vi "FTW-CodeGen-Prototype.vi"(0 "REPLACED_Connection":refnum<k24>, 2 "REPLACED_SQL Script":string, 5 "ADAPT_Data to Insert":T1(array[cluster]), 11 "REPLACED_error in":errorcluster) -> (4 "REPLACED_Connection out":refnum<k24>, 8 "REPLACED_Time to Execute":dbl format="%.6fsec", 10 "REPLACED_Number of Rows Inserted":i32, 15 "REPLACED_error out":errorcluster)   [LabVIEW 2015, in "FTW-dotNet-SQL-Insert.xnode"]
uses:
  FTW-dotNet-SQL-Insert.xnode
  System.Data
  src/error/FTW-ERR-ThrowError.vi
  src/error/FTW-ERR-CallChain.vi
  src/string/FTW-STR-ReplaceWhitespace.vi
  src/string/FTW-STR-Array-Delimit.vi
panel:
  # "Inputs"
  # "Outputs"
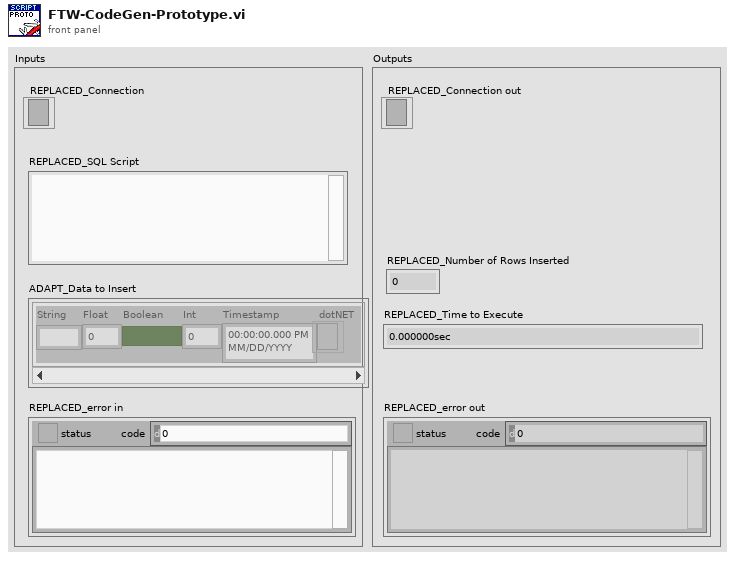
[diagram p1: front panel]
types:
  T1 = cluster{"String":string, "Float":dbl, "Boolean":bool, "Int":i64, "Timestamp":timestamp, "dotNET":refnum<k24>}[]
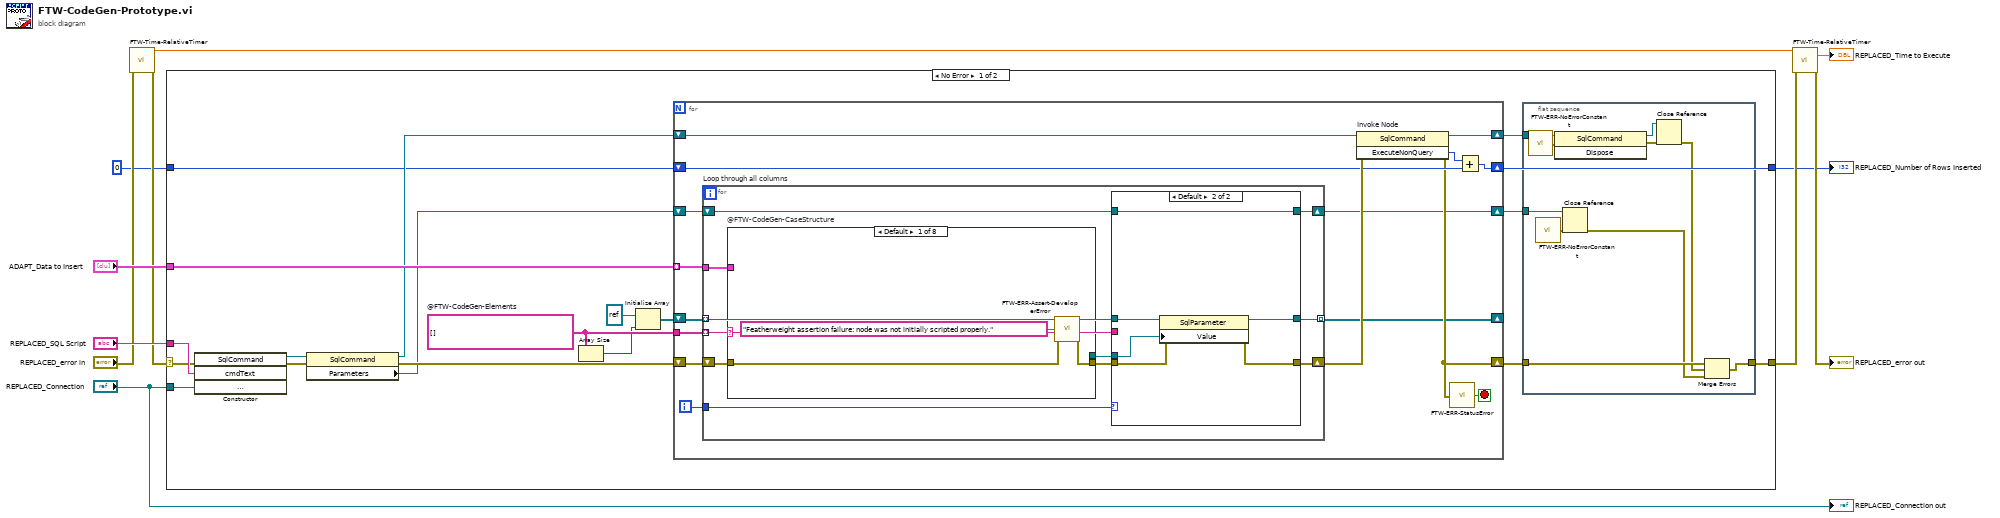
[diagram p0: block diagram]
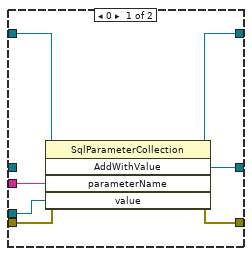
[diagram p2: hidden frame]
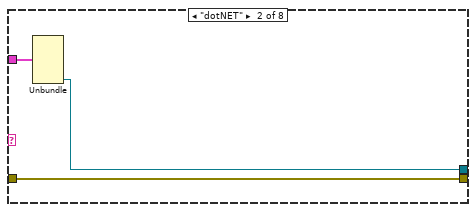
[diagram p3: hidden frame]
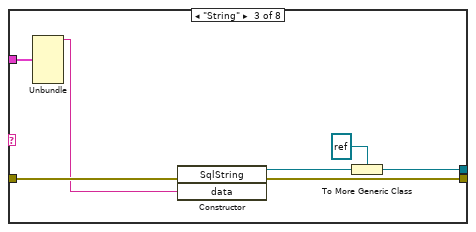
[diagram p4: hidden frame]
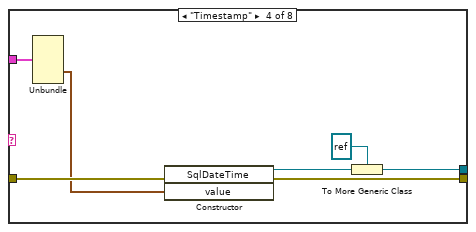
[diagram p5: hidden frame]
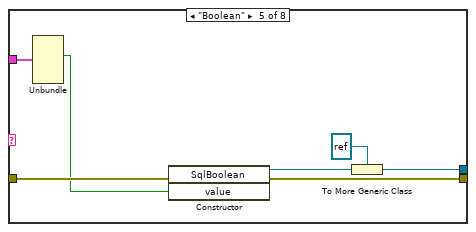
[diagram p6: hidden frame]
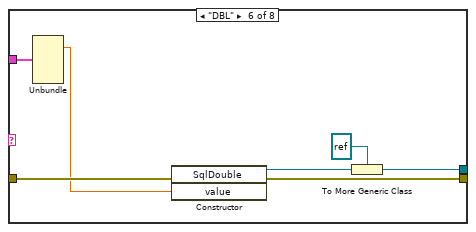
[diagram p7: hidden frame]
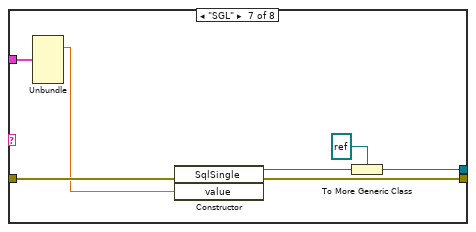
[diagram p8: hidden frame]
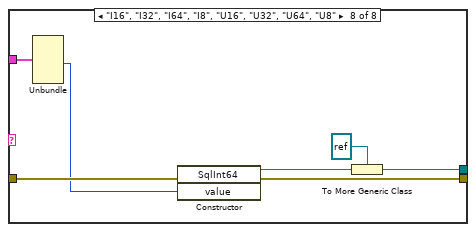
[diagram p9: hidden frame]
diagram:
  n1 = call "FTW-Time-RelativeTimer.vi"("error in"="REPLACED_error in") -> ("Current Timer Value"=w6:dbl, "error out"=w9:errorcluster)  [unwired: 12 in, 1 out]
  n2 = case shown="No Error" w9 {
    selector: w9 -> [w14 w130]
    tunnel: "REPLACED_SQL Script" -> [w15 _]
    tunnel: [w16 w130] -> w7
    tunnel: "ADAPT_Data to Insert" -> [w30 _]
    tunnel: "REPLACED_Connection" -> [w29 _]
    tunnel: [w23 w129] -> w4
    tunnel: 0 -> [w21 w129]
    frame No Error {
      w19 = string[] []  # @FTW-CodeGen-Elements
      n3 = constructor class="SqlCommand"(error in=w14, "cmdText"=w15, "connection"=w29) -> (reference out=w27:refnum<k24>, error out=w28:errorcluster)  [unwired: 2 in, 3 out]
      n4 = property class="SqlCommand"(reference=w27, error in=w28) -> (reference out=w25:refnum<k24>, error out=w26:errorcluster, "Parameters"=w13:refnum<k24>)
      n5 = Array Size(array=w19) -> (size(s)=w18:i32)
      n6 = Initialize Array(refnum<k24> refnum ("AddWithValue"), w18) -> (w17:refnum<k24>[])
      n7 = for {
        tunnel: w30 -> [w46] mode=indexing
        tunnel: w19 -> [w45]
        shift-right: [w37] -> w22
        shift-left: w26 -> [w44]
        shift-right: [w31] -> w24
        shift-left: w25 -> [w42]
        shift-right: [w38] -> w23
        shift-left: w21 -> [w40]
        shift-right: [w35] -> _
        shift-left: w17 -> [w33]
        shift-right: [w32] -> w12
        shift-left: w13 -> [w43]
        i -> [w34]
        stop <- w36 stop-if-true
        n8 = for "Loop through all columns" {
          shift-right: [w50] -> w41
          shift-left: w44 -> [w56]
          tunnel: w45 -> [w53] mode=indexing
          tunnel: w46 -> [w57]
          tunnel: [w48] -> w35 mode=indexing
          tunnel: w34 -> [w55]
          tunnel: w33 -> [w49] mode=indexing
          shift-right: [w47] -> w32
          shift-left: w43 -> [w52]
          n9 = case "@FTW-CodeGen-CaseStructure" shown="Default" w53 {
            tunnel: w56 -> [w73 w75 w83 w90 w97 w104 w111 w118]
            tunnel: [w72 w75 w77 w87 w94 w98 w105 w112] -> w54
            tunnel: w57 -> [_ w76 w82 w89 w96 w103 w110 w117]
            tunnel: [_ w74 w78 w84 w91 w99 w106 w113] -> w51
            frame Default {
              n10 = call "FTW-ERR-Assert-DeveloperError.vi"("Reason this error should never happen"="Featherweight assertion failure: node was not initially scripted properly.", "error in"=w73) -> ("error out"=w72:errorcluster)  [unwired: 13 in]
            }
            frame "dotNET" {
              n11 = Unbundle(w76) -> ("dotNET"=w74:refnum<k24>)  [unwired: 5 out]
            }
            frame "String" {
              n12 = Unbundle(w82) -> ("String"=w81:string)  [unwired: 5 out]
              n13 = constructor class="SqlString"(error in=w83, "data"=w81) -> (reference out=w79:refnum<k24>, error out=w77:errorcluster)  [unwired: 2 in, 2 out]
              n14 = To More Generic Class(target class=refnum<k24> refnum, reference=w79) -> (generic class reference=w78:refnum<k24>)
            }
            frame "Timestamp" {
              n15 = Unbundle(w89) -> ("Timestamp"=w88:timestamp)  [unwired: 5 out]
              n16 = constructor class="SqlDateTime"(error in=w90, "value"=w88) -> (reference out=w85:refnum<k24>, error out=w87:errorcluster)  [unwired: 2 in, 2 out]
              n17 = To More Generic Class(target class=refnum<k24> refnum, reference=w85) -> (generic class reference=w84:refnum<k24>)
            }
            frame "Boolean" {
              n18 = Unbundle(w96) -> ("Boolean"=w95:bool)  [unwired: 5 out]
              n19 = constructor class="SqlBoolean"(error in=w97, "value"=w95) -> (reference out=w92:refnum<k24>, error out=w94:errorcluster)  [unwired: 2 in, 2 out]
              n20 = To More Generic Class(target class=refnum<k24> refnum ("dotNET"), reference=w92) -> (generic class reference=w91:refnum<k24>)
            }
            frame "DBL" {
              n21 = Unbundle(w103) -> ("Float"=w102:dbl)  [unwired: 5 out]
              n22 = constructor class="SqlDouble"(error in=w104, "value"=w102) -> (reference out=w100:refnum<k24>, error out=w98:errorcluster)  [unwired: 2 in, 2 out]
              n23 = To More Generic Class(target class=refnum<k24> refnum ("dotNET"), reference=w100) -> (generic class reference=w99:refnum<k24>)
            }
            frame "SGL" {
              n24 = Unbundle(w110) -> ("Float"=w109:dbl)  [unwired: 5 out]
              n25 = constructor class="SqlSingle"(error in=w111, "value"=w109) -> (reference out=w107:refnum<k24>, error out=w105:errorcluster)  [unwired: 2 in, 2 out]
              n26 = To More Generic Class(target class=refnum<k24> refnum ("dotNET"), reference=w107) -> (generic class reference=w106:refnum<k24>)
            }
            frame "I16", "I32", "I64", "I8", "U16", "U32", "U64", "U8" {
              n27 = Unbundle(w117) -> ("Int"=w116:i64)  [unwired: 5 out]
              n28 = constructor class="SqlInt64"(error in=w118, "value"=w116) -> (reference out=w114:refnum<k24>, error out=w112:errorcluster)  [unwired: 2 in, 2 out]
              n29 = To More Generic Class(target class=refnum<k24> refnum ("dotNET"), reference=w114) -> (generic class reference=w113:refnum<k24>)
            }
          }
          n30 = case shown="Default" w55 {
            tunnel: w53 -> [w64 _]
            tunnel: w52 -> [w63 w65]
            tunnel: w54 -> [w62 w69]
            tunnel: w51 -> [w61 w68]
            tunnel: [w60 w67] -> w48
            tunnel: [w59 w70] -> w50
            tunnel: w49 -> [_ w66]
            tunnel: [w58 w65] -> w47
            frame 0 {
              n31 = invoke class="SqlParameterCollection" method="AddWithValue"(reference=w63, error in=w62, "parameterName"=w64, "value"=w61) -> (reference out=w58:refnum<k24>, error out=w59:errorcluster, "AddWithValue"=w60:refnum<k24>)  [unwired: 1 in, 2 out]
            }
            frame Default {
              n32 = property class="SqlParameter"(reference=w66, error in=w69, "Value"=w68) -> (reference out=w67:refnum<k24>, error out=w70:errorcluster)
            }
          }
        }
        n33 = invoke on="Invoke Node" class="SqlCommand" method="ExecuteNonQuery"(reference=w42, error in=w41) -> (reference out=w31:refnum<k24>, error out=w37:errorcluster, "ExecuteNonQuery"=w39:i32)  [unwired: 1 in]
        n34 = call "FTW-ERR-StatusError.vi"("error to check"=w37) -> ("Error?"=w36:bool)
        n35 = Add(x=w39, y=w40) -> (x+y=w38:i32)
      }
      n36 = flat-sequence {
        tunnel: w12 -> [w128]
        tunnel: w24 -> [w123]
        tunnel: w22 -> [w122]
        tunnel: [w121] -> w16
        frame #0 {
          n37 = call "FTW-ERR-NoErrorConstant.vi"() -> ("no error"=w124:errorcluster)
          n38 = call "FTW-ERR-NoErrorConstant.vi"() -> ("no error"=w127:errorcluster)
          n39 = invoke class="SqlCommand" method="Dispose"(reference=w123, error in=w124) -> (reference out=w125:refnum<k24>, error out=w126:errorcluster)  [unwired: 1 in, 1 out]
          n40 = Close Reference(reference=w128, error in (no error)=w127) -> (error out=w119:errorcluster)
          n41 = Close Reference(reference=w125, error in (no error)=w126) -> (error out=w120:errorcluster)
          n42 = Merge Errors(w122, w120, w119) -> (w121:errorcluster)
        }
      }
    }
    frame Error {
    }
  }
  "REPLACED_Number of Rows Inserted" <- w4
  n43 = call "FTW-Time-RelativeTimer.vi"("Previous Timer Value"=w6, "error in"=w7) -> ("Elapsed Time"=→"REPLACED_Time to Execute":dbl, "error out"=→"REPLACED_error out":errorcluster)  [unwired: 11 in, 1 out]
  "REPLACED_Connection out" <- "REPLACED_Connection"
